vi "Library_Error_init.vi"(8 "error in (no error)":errorcluster) -> (0 "error out":errorcluster)   [LabVIEW 2013]
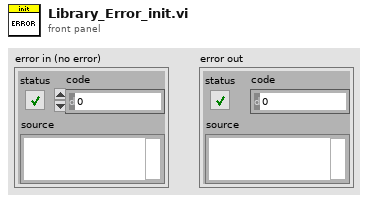
[diagram p1: front panel]
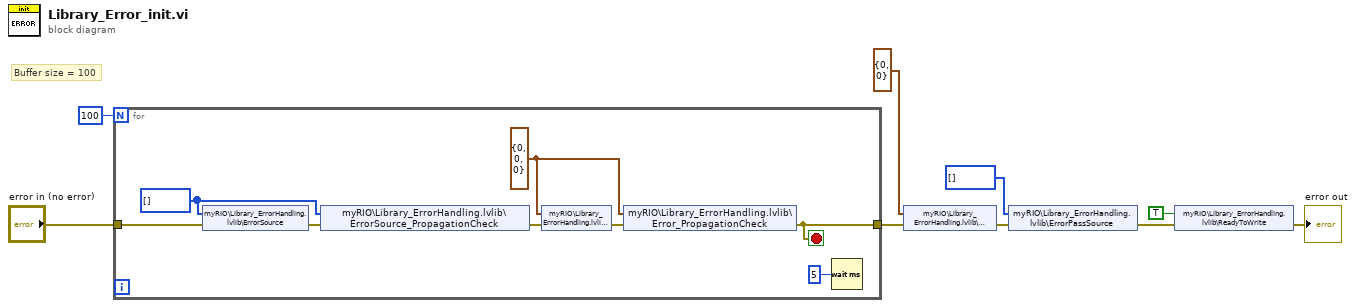
[diagram p0: block diagram]
diagram:
  # "Buffer size = 100"
  n1 = for {
    N: 100 -> [_]
    tunnel: [w10] -> w8
    tunnel: "error in (no error)" -> [w16]
    stop <- w10 stop-if-true
    w15 = u8[] [] ("ErrorSource")
    w14 = cluster{"Code":i32, "Priority":i32, "Class":i32} {"Code"=0, "Priority"=0, "Class"=0} ("Error")
    n2 = shared-variable "myRIO\\Library_ErrorHandling.lvlib\\ErrorSource"(w15, error in=w16) -> (error out=w13:errorcluster)
    n3 = shared-variable "myRIO\\Library_ErrorHandling.lvlib\\ErrorSource_PropagationCheck"(w15, error in=w13) -> (error out=w12:errorcluster)
    n4 = shared-variable "myRIO\\Library_ErrorHandling.lvlib\\Error"(w14, error in=w12) -> (error out=w11:errorcluster)
    n5 = shared-variable "myRIO\\Library_ErrorHandling.lvlib\\Error_PropagationCheck"(w14, error in=w11) -> (error out=w10:errorcluster)
    n6 = Wait (ms)(milliseconds to wait=u32 5) -> ()  [unwired: 1 out]
  }
  n7 = shared-variable "myRIO\\Library_ErrorHandling.lvlib\\ErrorPass"(cluster{"Code":i32, "Class":i32} {"Code"=0, "Class"=0} ("ErrorPass"), error in=w8) -> (error out=w3:errorcluster)
  n8 = shared-variable "myRIO\\Library_ErrorHandling.lvlib\\ErrorPassSource"(u8[] [] ("ErrorPassSource"), error in=w3) -> (error out=w4:errorcluster)
  n9 = shared-variable "myRIO\\Library_ErrorHandling.lvlib\\ReadyToWrite"(TRUE ("ReadyToWrite"), error in=w4) -> (error out=→"error out":errorcluster)
